vi "Call Function.vi"(8 "error in":errorcluster, 9 "arguments":string, 10 "function name":string, 11 "spark reference in":T1) -> (0 "error out":errorcluster, 2 "function response":T4, 3 "spark reference out":T1)   [LabVIEW 2013, in "Spark API.lvlib"]
doc: "Calls a Spark registered function (or web method) on a connected Spark device."
uses:
  Spark API.lvlib
  Controls/Spark Reference.ctl
  <vilib>/httpClient/ClientHandle.ctl
  Controls/Device Query JSON.ctl
  Controls/Function Response JSON.ctl
  <vilib>/httpClient/POSTBuffer.vi
  <vilib>/httpClient/LabVIEWHTTPClient.lvlib
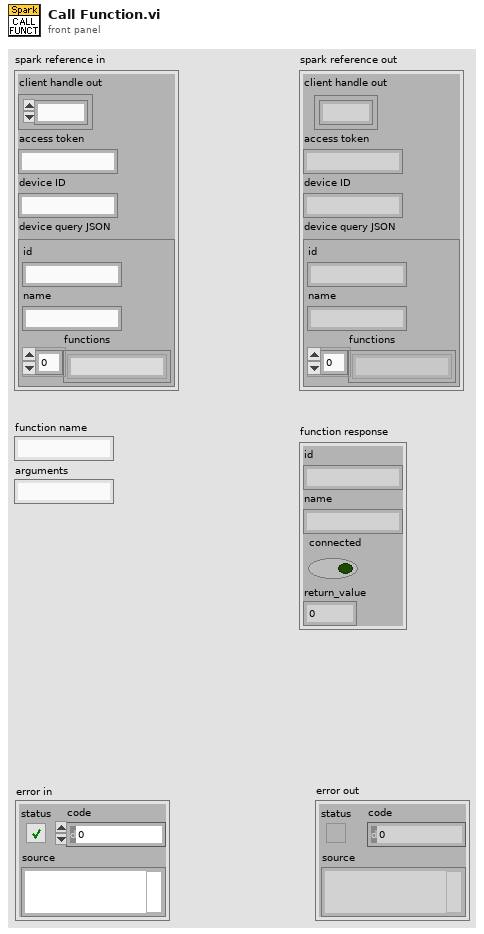
[diagram p1: front panel]
types:
  T1 = typedef "Spark API.lvlib/Spark Reference.ctl" = cluster{"client handle out":T2, "access token":string, "device ID":string, "device query JSON":T3}
  T2 = typedef "LabVIEWHTTPClient.lvlib/ClientHandle.ctl" = refnum<k1>
  T3 = typedef "Spark API.lvlib/Device Query JSON.ctl" = cluster{"id":string, "name":string, "functions":string[]}
  T4 = typedef "Spark API.lvlib/Function Response JSON.ctl" = cluster{"id":string, "name":string, "connected":bool, "return_value":dbl}
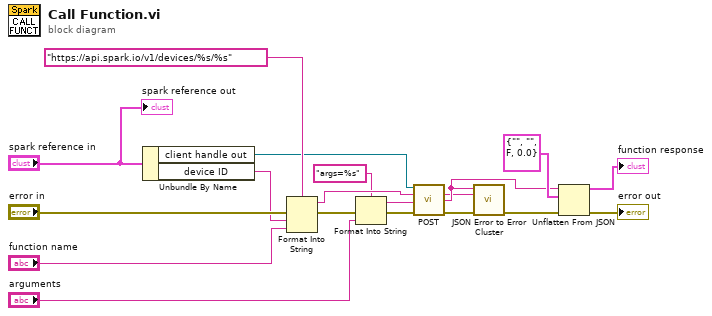
[diagram p0: block diagram]
diagram:
  n1 = Unbundle By Name("spark reference in") -> ("client handle out"=w14:T2, "device ID"=w13:string)
  n2 = Format Into String(format string="https://api.spark.io/v1/devices/%s/%s" ("url"), error in="error in", w13, "function name") -> (resulting string=w18:string, error out=w6:errorcluster)  [unwired: 1 in]
  n3 = Format Into String(format string="args=%s", error in=w6, "arguments") -> (resulting string=w9:string, error out=w5:errorcluster)  [unwired: 1 in]
  n4 = call-poly <vilib>:"POST.vi"("client handle"=w14, "url"=w18, "buffer"=w9, "error in (no error)"=w5) -> ("headers"=w2:string, "body"=w3:string, "error out"=w8:errorcluster)  [unwired: 8 in, 1 out]
  n5 = call "JSON Error to Error Cluster.vi"("error in (no error)"=w8, "headers"=w2, "JSON string"=w3) -> ("error out"=w4:errorcluster)  [unwired: 8 in]
  n6 = Unflatten From JSON(JSON string=w3, type and defaults=T4 {"id"="", "name"="", "connected"=FALSE, "return_value"=0.0} ("Function Response"), error in (no error)=w4) -> (value=→"function response":T4, error out=→"error out":errorcluster)  [unwired: 4 in]
  "spark reference out" <- "spark reference in"
